vi "ChipKit Character LCD.vi"() -> ()   [LabVIEW 2011, in "LabVIEW Interface for ChipKit.lvlib"]
doc: "Writes the text on the front panel to the LCD Screen using 4-bit mode."
uses:
  <vilib>/LabVIEW Interface for ChipKit/LabVIEW Interface for ChipKit.lvlib
  <vilib>/LabVIEW Interface for ChipKit/Private/Type Defs/LCD Pin Config 4-bit.ctl
  <vilib>/LabVIEW Interface for ChipKit/Private/Type Defs/Chipkit Resource.ctl
  <vilib>/LabVIEW Interface for ChipKit/Private/Type Defs/Board Type.ctl
  <vilib>/LabVIEW Interface for ChipKit/Private/Type Defs/Connection Type.ctl
panel:
  in  "LCD Text":string
  in  "Columns":u8
  in  "Rows":u8
  in  "ChipKit Configuration":T1={"COM Port"="", "Board Type"=enum."ChipKit Uno32", "Connection Type"=enum."USB / Serial", "Baud Rate (115200)"=115200, "Bytes Per Packet (15)"=15}
  in  "LCD Pin Config 4 Bit":T4={"RS"=12, "RW"=255, "Enable"=11, "D4"=5, "D5"=4, "D6"=3, "D7"=2, "LCD"=10}
  # "Character LCD Example\n\nThis example demonstrates how to read a single analog input value from the chipkit and display the value on a waveform chart.\n\nInstructions\n1. Select the COM Port associated with the ChipKit.\n2. Select the Board Type.\n3. Select the LCD RS, RW, Enable, and D4-D7 Pins.\n4. Enter text to write to the LCD in the LCD Text control.\n4. Click the Run Arrow."
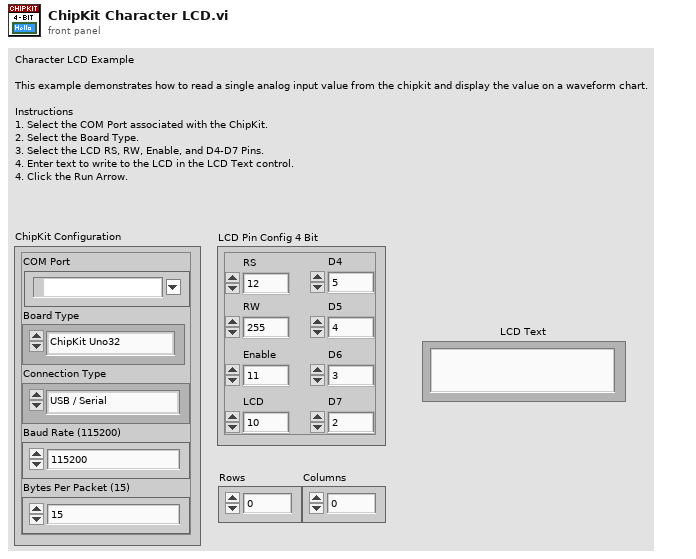
[diagram p1: front panel]
types:
  T1 = typedef "LabVIEW Interface for ChipKit.lvlib/Chipkit Resource.ctl" = cluster{"COM Port":refnum<visa-resource-name>, "Board Type":T2, "Connection Type":T3, "Baud Rate (115200)":u32, "Bytes Per Packet (15)":u32}
  T2 = typedef "LabVIEW Interface for ChipKit.lvlib/Board Type.ctl" = enum16{"ChipKit uC32", "ChipKit Uno32", "ChipKit Max32"}
  T3 = typedef "LabVIEW Interface for ChipKit.lvlib/Connection Type.ctl" = enum8{"USB / Serial", "XBEE", "BlueSmirf (Bluetooth)"}
  T4 = typedef "LabVIEW Interface for ChipKit.lvlib/LCD Pin Config 4-bit.ctl" = cluster{"RS":u8, "RW":u8, "Enable":u8, "D4":u8, "D5":u8, "D6":u8, "D7":u8, "LCD":u8}
  T5 = enum8{"String", "Binary", "Decimal", "Octal", "Hexadecimal"}
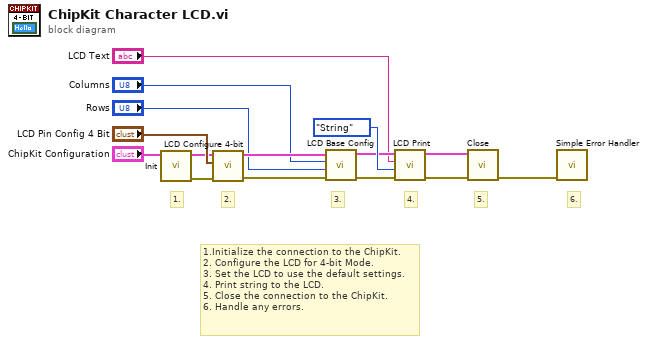
[diagram p0: block diagram]
diagram:
  # "6."
  # "1.Initialize the connection to the ChipKit.\n2. Configure the LCD for 4-bit Mode.\n3. Set the LCD to use the default settings.\n4. Print string to the LCD.\n5. Close the connection to the ChipKit.\n6. Handle any errors."
  # "5."
  # "4."
  # "3."
  # "2."
  # "1."
  n1 = call <vilib>:"Init.vi"("ChipKit Configuration"="ChipKit Configuration") -> ("Error Out"=w8:errorcluster, "ChipKit Configuration"=w6:T1)  [unwired: 9 in]
  n2 = call <vilib>:"LCD Configure 4-bit.vi"("Error In"=w8, "LCD Pin Config 4 Bit"="LCD Pin Config 4 Bit", "ChipKit Resource"=w6) -> ("Error Out"=w9:errorcluster, "ChipKit Resource"=w5:T1)  [unwired: 7 in]
  n3 = call <vilib>:"LCD Base Config.vi"("Error In"=w9, "Rows"="Rows", "Columns"="Columns", "ChipKit Resource"=w5) -> ("Error Out"=w10:errorcluster, "ChipKit Resource"=w11:T1)  [unwired: 6 in]
  n4 = call <vilib>:"LCD Print.vi"("Error In"=w10, "Base (String)"=T5."String", "Data"="LCD Text", "ChipKit Resource"=w11) -> ("Error Out"=w13:errorcluster, "ChipKit Resource"=w14:T1)  [unwired: 6 in]
  n5 = call <vilib>:"Close.vi"("Error In"=w13, "ChipKit Configuration"=w14) -> ("Error Out"=w12:errorcluster)  [unwired: 9 in]
  n6 = call <vilib>:"Simple Error Handler.vi"("error in (no error)"=w12) -> ()  [unwired: 4 in, 5 out]
